vi "Variable URL from PSP URL.vi"(8 "error in (no error)":errorcluster, 11 "PSP URL":string) -> (0 "error out":errorcluster, 3 "Shared Variable URL":refnum<k21>)   [LabVIEW 2024]
doc: "Converts a PSP URL to a shared variable URL."
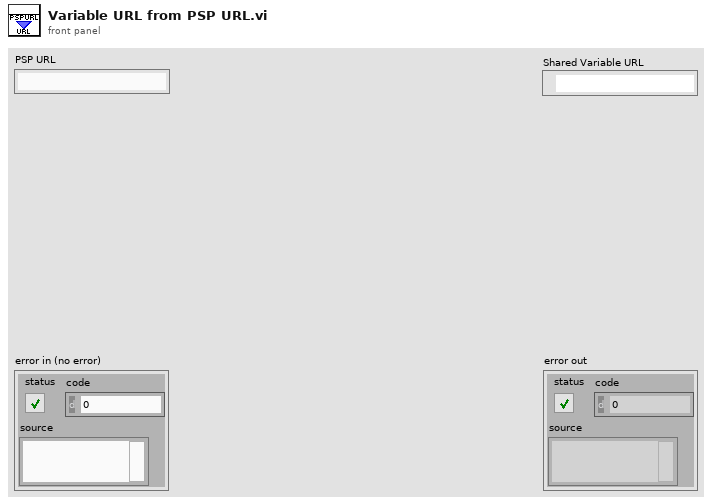
[diagram p1: front panel]
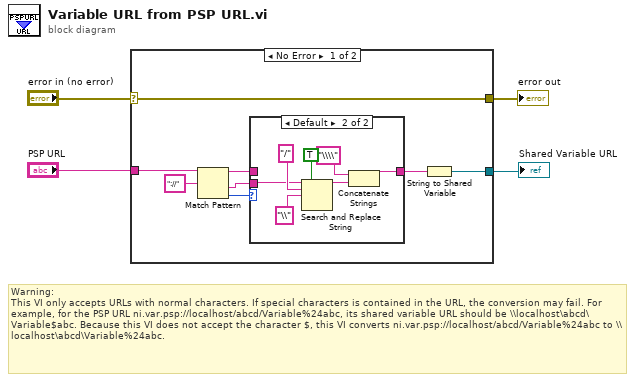
[diagram p0: block diagram]
diagram:
  # "Warning: \nThis VI only accepts URLs with normal characters. If special characters is contained in the URL, the conversion may fail. For example, for the PSP URL ni.var.psp://localhost/abcd/Variable%24abc, its shared variable URL should be \\\\localhost\\abcd\\Variable$abc. Because this VI does not accept the character $, this VI converts ni.var.psp://localhost/abcd/Variable%24abc to \\\\localhost\\abcd\\Variable%24abc."
  n1 = case shown="No Error" "error in (no error)" {
    selector: "error in (no error)" -> [w5 w21]
    tunnel: [w5 w21] -> w3
    tunnel: "PSP URL" -> [w7 _]
    tunnel: [w6 _] -> w2
    frame No Error {
      n2 = Match Pattern(string=w7, regular expression="://" ("format string")) -> (before substring=w12:string, after substring=w9:string, offset past match=w11:i32)  [unwired: 1 in, 1 out]
      n3 = case shown="Default" w11 {
        tunnel: w9 -> [_ w15]
        tunnel: w12 -> [w13 _]
        tunnel: [w13 w14] -> w8
        frame -1 {
        }
        frame Default {
          n4 = Search and Replace String(replace all?=TRUE ("replace all? (F)"), input string=w15, search string="/", replace string="\\" ("replace string (\"\")")) -> (result string=w17:string)  [unwired: 4 in, 3 out]
          n5 = Concatenate Strings("\\\\" ("string"), w17) -> (w14:string)
        }
      }
      n6 = String to Shared Variable(0:w8) -> (2:w6:refnum<k21>)  [unwired: 1 out]
    }
    frame Error {
    }
  }
  "error out" <- w3
  "Shared Variable URL" <- w2
